vi "test3.1-MappingRelationshipByExternalRegistration_API.vi"(8 "error in (no error)":errorcluster, 11 "TestCase in":refnum<class "testcase-CSMBroadcast.lvclass">) -> (0 "error out":errorcluster, 3 "TestCase out":refnum<class "testcase-CSMBroadcast.lvclass">)   [LabVIEW 2017, in "testcase-CSMBroadcast.lvclass"]
uses:
  testcase-CSMBroadcast.lvclass
  src/user.lib/_NEVSTOP/Communicable State Machine(CSM)/Communicable State Machine.lvlib
  <vilib>/addons/_JKI Toolkits/VI Tester/TestCase.llb/TestCase.lvclass
  CSM/CSM-Testcase.lvlib
  C:/Program Files (x86)/National Instruments/LabVIEW 2017/vi.lib/addons/_JKI Toolkits/VI Tester/TestCase.llb/TestCase.lvclass
panel:
  out "Loop Count":i32
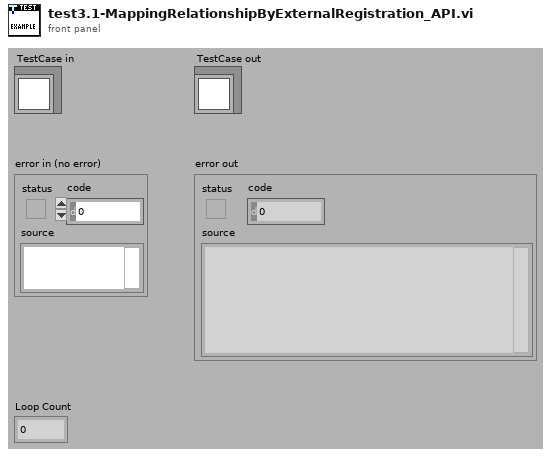
[diagram p1: front panel]
types:
  T1 = cluster{"Status":string, "Source CSM":string, "Target CSM":string, "Target API":string}[]
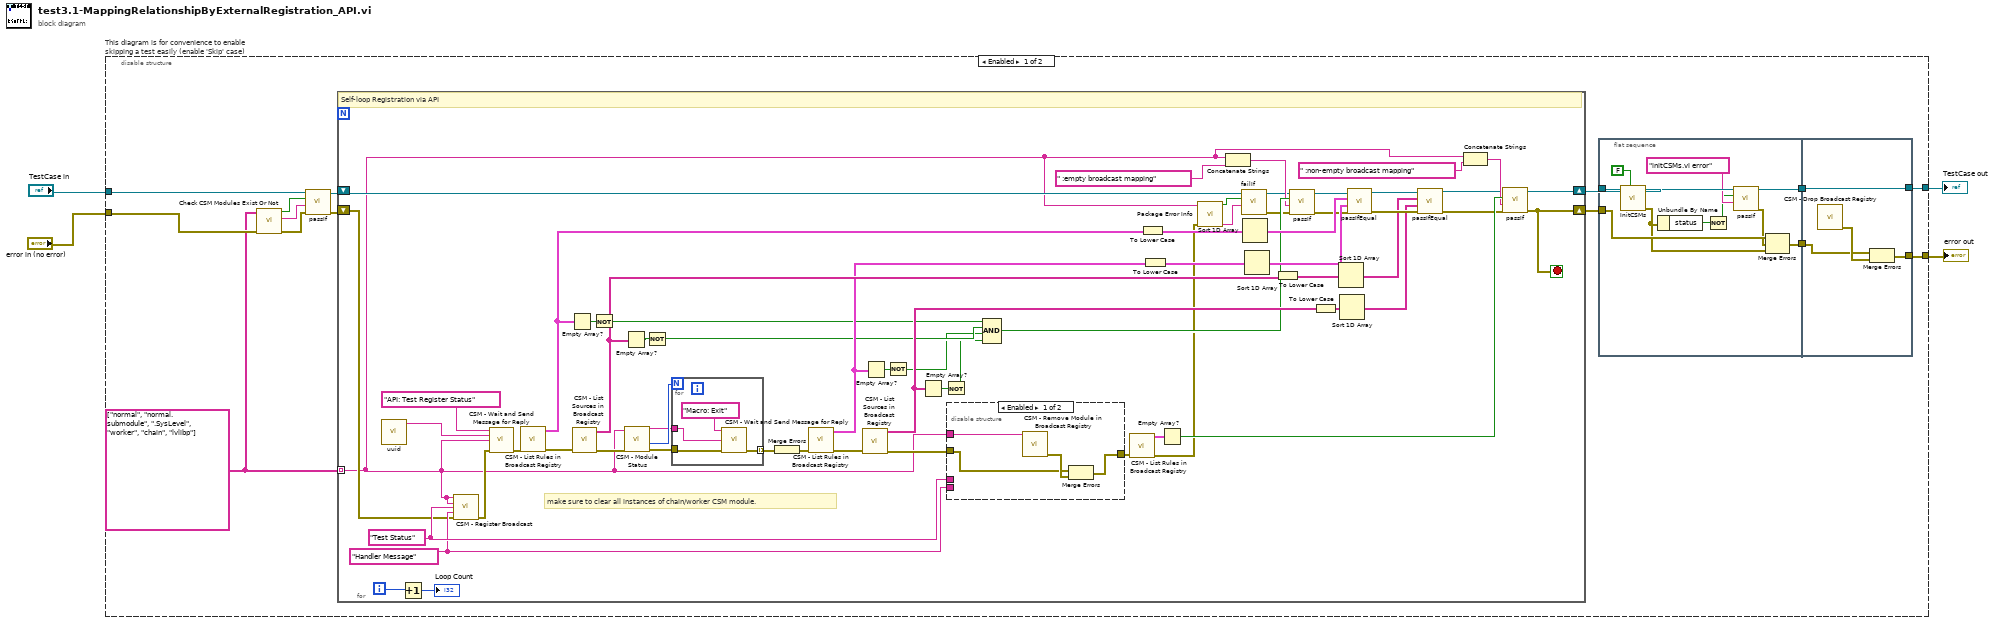
[diagram p0: block diagram]
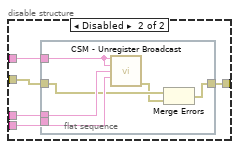
[diagram p2: hidden frame]
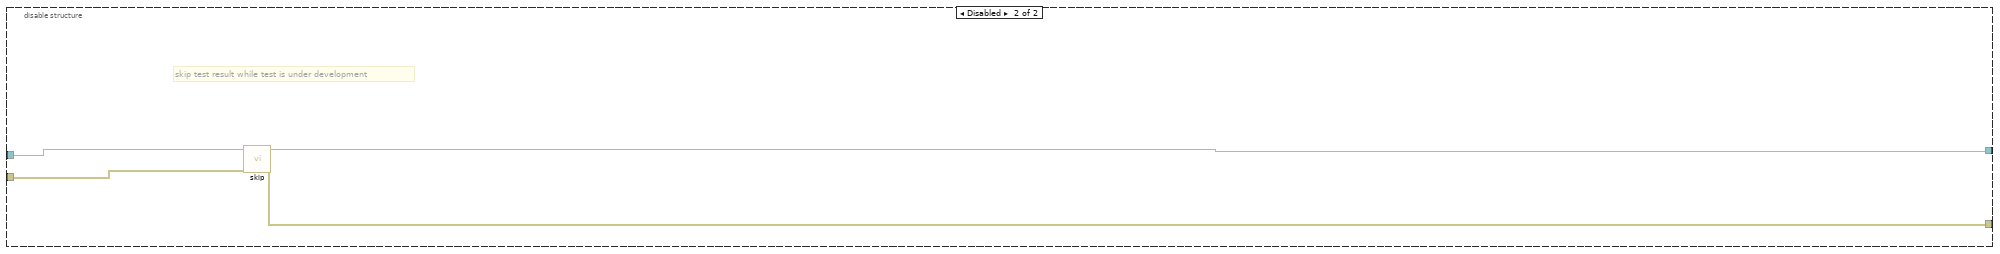
[diagram p3: hidden frame]
diagram:
  n1 = disable-structure "This diagram is for convenience to enable skipping a test easily (enable 'Skip' case)" shown="Enabled" {
    disable-tunnel: "TestCase in" -> [w12 w117]
    disable-tunnel: [w7 w115] -> w1
    disable-tunnel: [w6 w116] -> w3
    disable-tunnel: "error in (no error)" -> [w10 w114]
    frame Enabled {
      w8 = string[] ["normal", "normal.submodule", ".SysLevel", "worker", "chain", "lvlibp"]
      n2 = call "Check CSM Modules Exist Or Not.vi"("error in"=w10, "CSM names in"=w8) -> ("error out"=w13:errorcluster, "Debug string"=w14:string, "All Modules Exist?"=w15:bool)  [unwired: 7 in]
      n3 = call-dynamic "passIf.vi"("error in (no error)"=w13, "message (\"\")"=w14, "pass"=w15, "TestCase in"=w12) -> ("error out"=w9:errorcluster, "TestCase out"=w11:refnum<class "testcase-CSMBroadcast.lvclass">)  [unwired: 6 in]
      n4 = for {
        tunnel: w8 -> [w34] mode=indexing
        shift-right: [w59] -> w17
        shift-left: w11 -> [w38]
        shift-right: [w57] -> w16
        shift-left: w9 -> [w45]
        i -> [w79]
        stop <- w57 stop-if-true
        w62 = "Handler Message" ("Response Message (If \"\", Same as Source Message)")
        w63 = "Test Status" ("Status")
        # "make sure to clear all instances of chain/worker CSM module."
        # "Self-loop Registration via API"
        n5 = call "uuid.vi"() -> ("UUID"=w93:string)  [unwired: 11 in]
        n6 = Increment(x=w79) -> (x+1=→"Loop Count":i32)
        n7 = call "CSM - Register Broadcast.vi"("CSM Name(Empty for Broadcast Event)"=w34, "Source CSM Name (* as Default)"=w34, "Trigger"=w63, "API (If \"\", Same as Trigger)"=w62, "Error In"=w45) -> ("error out"=w64:errorcluster)  [unwired: 9 in, 1 out]
        n8 = call "CSM - Wait and Send Message for Reply.vi"("State"="API: Test Register Status", "Arguments (\"\")"=w93, "Target Module"=w34, "Error In (No Error)"=w64) -> ("error out"=w92:errorcluster)  [unwired: 8 in, 3 out]
        n9 = call "CSM - List Rules in Broadcast Registry.vi"("error in (no error)"=w92) -> ("error out"=w91:errorcluster, "Rule Entries"=w77:T1)  [unwired: 8 in, 1 out]
        n10 = Empty Array?(array=w77) -> (empty?=w76:bool)
        n11 = call "CSM - List Sources in Broadcast Registry.vi"("error in (no error)"=w91) -> ("error out"=w54:errorcluster, "Broadcast Names"=w74:string[])  [unwired: 9 in]
        n12 = Not(x=w76) -> (.not. x?=w69:bool)
        n13 = Empty Array?(array=w74) -> (empty?=w75:bool)
        n14 = call "CSM - Module Status.vi"("Error In"=w54, "CSM Name"=w34) -> ("error out"=w53:errorcluster, "#Nodes"=w56:i32, "CSM Name (Dup)"=w55:string)  [unwired: 5 in, 2 out]
        n15 = Not(x=w75) -> (.not. x?=w68:bool)
        n16 = for {
          N: w56 -> [_]
          tunnel: w55 -> [w97]
          tunnel: w53 -> [w96]
          tunnel: [w95] -> w51 mode=indexing
          n17 = call "CSM - Wait and Send Message for Reply.vi"("State"="Macro: Exit", "Target Module"=w97, "Error In (No Error)"=w96) -> ("error out"=w95:errorcluster)  [unwired: 9 in, 3 out]
        }
        n18 = Merge Errors(w51) -> (w52:errorcluster)
        n19 = call "CSM - List Rules in Broadcast Registry.vi"("error in (no error)"=w52) -> ("error out"=w90:errorcluster, "Rule Entries"=w72:T1)  [unwired: 8 in, 1 out]
        n20 = call "CSM - List Sources in Broadcast Registry.vi"("error in (no error)"=w90) -> ("error out"=w65:errorcluster, "Broadcast Names"=w70:string[])  [unwired: 9 in]
        n21 = Empty Array?(array=w72) -> (empty?=w73:bool)
        n22 = Not(x=w73) -> (.not. x?=w67:bool)
        n23 = Empty Array?(array=w70) -> (empty?=w71:bool)
        n24 = Not(x=w71) -> (.not. x?=w66:bool)
        n25 = disable-structure shown="Enabled" {
          disable-tunnel: w65 -> [w99 w104]
          disable-tunnel: [w100 w103] -> w61
          disable-tunnel: w34 -> [w101 w105]
          disable-tunnel: w63 -> [_ w107]
          disable-tunnel: w62 -> [_ w106]
          frame Enabled {
            n26 = call "CSM - Remove Module in Broadcast Registry.vi"("CSM Name"=w101) -> ("error out"=w102:errorcluster)  [unwired: 13 in, 1 out]
            n27 = Merge Errors(w99, w102) -> (w100:errorcluster)
          }
          frame Disabled {
            n28 = flat-sequence {
              tunnel: w107 -> [w113]
              tunnel: w106 -> [w112]
              tunnel: w105 -> [w111]
              tunnel: w104 -> [w110]
              tunnel: [w108] -> w103
              frame #0 {
                n29 = call "CSM - Unregister Broadcast.vi"("CSM Name(Empty for Broadcast Event)"=w111, "Source CSM Name (* as Default)"=w111, "Trigger"=w113, "API (\"*\" as Default)"=w112) -> ("error out"=w109:errorcluster)  [unwired: 10 in, 1 out]
                n30 = Merge Errors(w110, w109) -> (w108:errorcluster)
              }
            }
          }
        }
        n31 = Compound Arithmetic op=AND(w69, w68, w67, w66) -> (w44:bool)
        n32 = call "CSM - List Rules in Broadcast Registry.vi"("error in (no error)"=w61) -> ("error out"=w35:errorcluster, "Rule Entries"=w60:T1)  [unwired: 8 in, 1 out]
        n33 = To Lower Case(string=w77) -> (all lower case string=w89:T1)
        n34 = To Lower Case(string=w72) -> (all lower case string=w88:T1)
        n35 = Empty Array?(array=w60) -> (empty?=w58:bool)
        n36 = call "Package Error Info.vi"("error in"=w35, "String in"=w34) -> ("packed error info out"=w39:string, "error status"=w40:bool)  [unwired: 8 in]
        n37 = Concatenate Strings(w34, " :empty broadcast mapping" ("string")) -> (w43:string)
        n38 = call-dynamic "failIf.vi"("message (\"\")"=w39, "fail"=w40, "TestCase in"=w38) -> ("error out"=w36:errorcluster, "TestCase out"=w37:refnum<class "testcase-CSMBroadcast.lvclass">)  [unwired: 7 in]
        n39 = Sort 1D Array(array=w89) -> (sorted array=w87:T1)
        n40 = Sort 1D Array(array=w88) -> (sorted array=w86:T1)
        n41 = To Lower Case(string=w74) -> (all lower case string=w83:string[])
        n42 = call-dynamic "passIf.vi"("error in (no error)"=w36, "message (\"\")"=w43, "pass"=w44, "TestCase in"=w37) -> ("error out"=w47:errorcluster, "TestCase out"=w46:refnum<class "testcase-CSMBroadcast.lvclass">)  [unwired: 6 in]
        n43 = To Lower Case(string=w70) -> (all lower case string=w82:string[])
        n44 = Sort 1D Array(array=w83) -> (sorted array=w81:string[])
        n45 = Sort 1D Array(array=w82) -> (sorted array=w80:string[])
        n46 = call-dynamic "passIfEqual.vi"("error in (no error)"=w47, "y"=w86, "x"=w87, "TestCase in"=w46) -> ("error out"=w84:errorcluster, "TestCase out"=w85:refnum<class "testcase-CSMBroadcast.lvclass">)  [unwired: 6 in]
        n47 = call-dynamic "passIfEqual.vi"("error in (no error)"=w84, "y"=w80, "x"=w81, "TestCase in"=w85) -> ("error out"=w41:errorcluster, "TestCase out"=w42:refnum<class "testcase-CSMBroadcast.lvclass">)  [unwired: 6 in]
        n48 = Concatenate Strings(w34, " :non-empty broadcast mapping" ("string")) -> (w48:string)
        n49 = call-dynamic "passIf.vi"("error in (no error)"=w41, "message (\"\")"=w48, "pass"=w58, "TestCase in"=w42) -> ("error out"=w57:errorcluster, "TestCase out"=w59:refnum<class "testcase-CSMBroadcast.lvclass">)  [unwired: 6 in]
      }
      n50 = flat-sequence {
        tunnel: w17 -> [w29]
        tunnel: [w26] -> w18
        tunnel: w16 -> [w23]
        tunnel: [w20] -> w5
        tunnel: w18 -> [w32]
        tunnel: [w32] -> w7
        tunnel: [w31] -> w6
        tunnel: w5 -> [w30]
        frame #0 {
          n51 = call "InitCSMs.vi"("Enable building lvlibp?"=FALSE, "testcase-CSMStatus in"=w29) -> ("error out"=w21:errorcluster, "testcase-CSMStatus out"=w27:refnum<class "testcase-CSMBroadcast.lvclass">)  [unwired: 8 in]
          n52 = Unbundle By Name(w21) -> ("status"=w25:bool)
          n53 = Not(x=w25) -> (.not. x?=w19:bool)
          n54 = call-dynamic "passIf.vi"("message (\"\")"="initCSMs.vi error" ("message (\"\")"), "pass"=w19, "TestCase in"=w27) -> ("error out"=w22:errorcluster, "TestCase out"=w26:refnum<class "testcase-CSMBroadcast.lvclass">)  [unwired: 7 in]
          n55 = Merge Errors(w23, w22, w21) -> (w20:errorcluster)
        }
        frame #1 {
          n56 = call "CSM - Drop Broadcast Registry.vi"() -> ("error out"=w33:errorcluster)  [unwired: 15 in]
          n57 = Merge Errors(w30, w33) -> (w31:errorcluster)
        }
      }
    }
    frame Disabled {
      # "skip test result while test is under development"
      n58 = call <vilib>:"skip.vi"("error in (no error)"=w114, "TestCase in"=w117) -> ("error out"=w116:errorcluster, "TestCase out"=w115:refnum<class "testcase-CSMBroadcast.lvclass">)  [unwired: 8 in]
    }
  }
  "error out" <- w3
  "TestCase out" <- w1
